vi "SMTP Email Send Message Start.vi"(4 "error in (no error)":errorcluster, 5 "return address":string, 6 "recipients":string[](array[string]), 7 "smtp session":T1) -> (0 "error out":errorcluster, 2 "invalid recipients":string[](array[string]), 3 "smtp session out":T1)   [LabVIEW 2012, in "NewNI_SMTPEmail.lvlib"]
uses:
  NewNI_SMTPEmail.lvlib
  SMTP Email Session.ctl
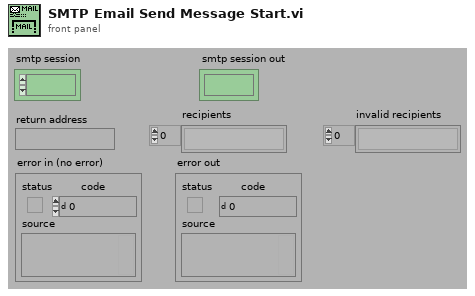
[diagram p1: front panel]
types:
  T1 = typedef "NewNI_SMTPEmail.lvlib/SMTP Email Session.ctl" = refnum<k1>
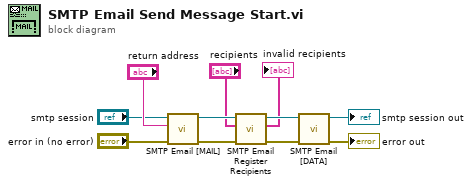
[diagram p0: block diagram]
diagram:
  n1 = call "SMTP Email [MAIL].vi"("error in (no error)"="error in (no error)", "return address"="return address", "smtp session"="smtp session") -> ("error out"=w9:errorcluster, "smtp session out"=w10:T1)  [unwired: 3 out]
  n2 = call "SMTP Email Register Recipients.vi"("error in (no error)"=w9, "recipients"="recipients", "smtp session"=w10) -> ("error out"=w11:errorcluster, "invalid recipients"=→"invalid recipients":string[], "smtp session out"=w8:T1)  [unwired: 1 in, 1 out]
  n3 = call "SMTP Email [DATA].vi"("error in (no error)"=w11, "smtp session"=w8) -> ("error out"=→"error out":errorcluster, "smtp session out"=→"smtp session out":T1)  [unwired: 1 in, 3 out]
